vi "Display Channel Datapath.vi"(0 "llp packet":T5, 1 "reset":bool, 2 "clear processing pipeline":bool, 3 "gate display until frame complete":bool, 5 "serial channel display parameters":T9, 7 "serial channel selector":fxp<+,3,3>, 9 "input valid":bool, 11 "display channel resources":T2, 12 "enable channel":bool) -> (4 "display channel status":T1, 6 "pending display frames":i8, 14 "ready for input":bool)   [LabVIEW 2020, in "GettingStarted_Common_148X_FPGA.lvlib"]
uses:
  GettingStarted_Common_148X_FPGA.lvlib
  <instrlib>/FlexRIO/CSI-2/v2/FPGA/Types/Display Parameters.ctl
  <instrlib>/FlexRIO/CSI-2/v2/Common/Types/LLP Data Type.ctl
  <instrlib>/FlexRIO/CSI-2/v2/FPGA/Types/LLP Packet.ctl
  <instrlib>/FlexRIO/CSI-2/v2/FPGA/Types/LLP Packet Header.ctl
  <instrlib>/FlexRIO/CSI-2/v2/FPGA/Types/LLP Packet Payload.ctl
  <instrlib>/FlexRIO/CSI-2/v2/FPGA/Types/LLP Packet Footer.ctl
  Types/Display Channel Resources.ctl
  Types/Serial Channel Resources.ctl
  Types/Single Serial Channel Resources.ctl
  Types/Display Channel Status.ctl
  Types/Image Metadata.ctl
  <instrlib>/FlexRIO/CSI-2/v2/FPGA/NI CSI-2 API FPGA v2.lvlib
  <instrlib>/FlexRIO/CSI-2/v2/Common/NI CSI-2 API Common v2.lvlib
  <instrlib>/_niInstr/Basic Elements/v1/FPGA/niInstr Basic Elements v1 FPGA.lvlib
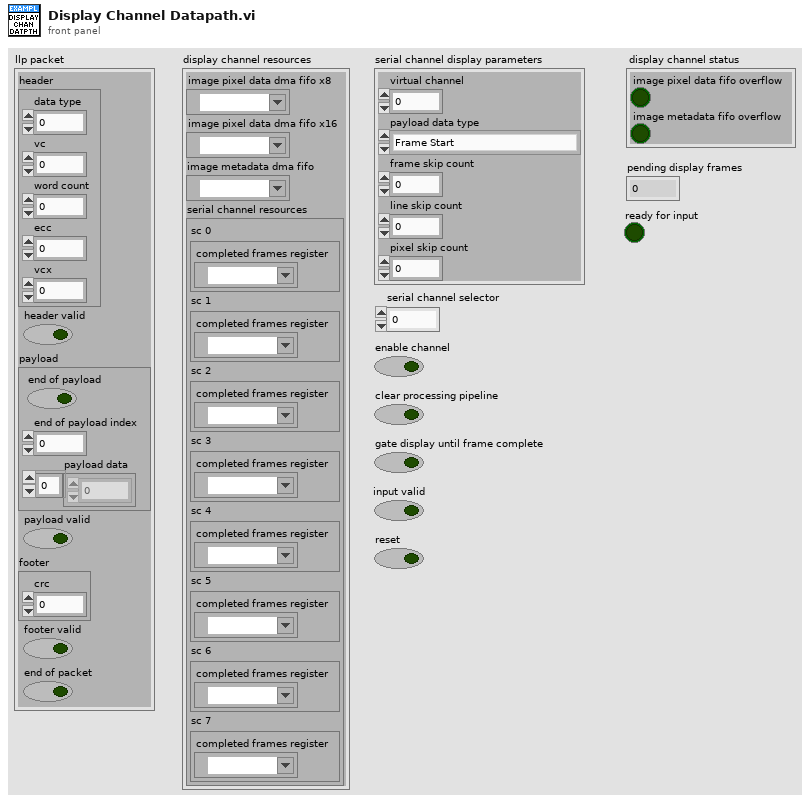
[diagram p1: front panel]
types:
  T1 = typedef "GettingStarted_Common_148X_FPGA.lvlib/Display Channel Status.ctl" = cluster{"image pixel data fifo overflow":bool, "image metadata fifo overflow":bool}
  T2 = typedef "GettingStarted_Common_148X_FPGA.lvlib/Display Channel Resources.ctl" = cluster{"image pixel data dma fifo x8":refnum<k21>, "image pixel data dma fifo x16":refnum<k21>, "image metadata dma fifo":refnum<k21>, "serial channel resources":T3}
  T3 = typedef "GettingStarted_Common_148X_FPGA.lvlib/Serial Channel Resources.ctl" = cluster{"sc 0":T4, "sc 1":T4, "sc 2":T4, "sc 3":T4, "sc 4":T4, "sc 5":T4, "sc 6":T4, "sc 7":T4}
  T4 = typedef "GettingStarted_Common_148X_FPGA.lvlib/Single Serial Channel Resources.ctl" = cluster{"completed frames register":refnum<k21>}
  T5 = typedef "NI CSI-2 API FPGA v2.lvlib/LLP Packet.ctl" = cluster{"header":T6, "header valid":bool, "payload":T7, "payload valid":bool, "footer":T8, "footer valid":bool, "end of packet":bool}
  T6 = typedef "NI CSI-2 API FPGA v2.lvlib/LLP Packet Header.ctl" = cluster{"word count":u16, "ecc":fxp<+,6,6>, "vcx":fxp<+,2,2>, "data type":fxp<+,6,6>, "vc":fxp<+,2,2>}
  T7 = typedef "NI CSI-2 API FPGA v2.lvlib/LLP Packet Payload.ctl" = cluster{"end of payload":bool, "end of payload index":fxp<+,3,3>, "payload data":u8[]}
  T8 = typedef "NI CSI-2 API FPGA v2.lvlib/LLP Packet Footer.ctl" = cluster{"crc":u16}
  T9 = typedef "NI CSI-2 API FPGA v2.lvlib/Display Parameters.ctl" = cluster{"virtual channel":fxp<+,4,4>, "payload data type":T10, "frame skip count":u16, "line skip count":u8, "pixel skip count":fxp<+,5,5>}
  T10 = typedef "NI CSI-2 API Common v2.lvlib/LLP Data Type.ctl" = enum8{"Frame Start", "Frame End", "Line Start", "Line End", "End of Transmission", "Reserved 0", "Reserved 1", "Reserved 2", "Generic Short Packet 1", "Generic Short Packet 2", "Generic Short Packet 3", "Generic Short Packet 4", "Generic Short Packet 5", "Generic Short Packet 6", "Generic Short Packet 7", "Generic Short Packet 8", "Null", "Blanking Data", "Embedded 8-bit non Image Data", "Generic Long Packet 1", "Generic Long Packet 2", "Generic Long Packet 3", "Generic Long Packet 4", "Reserved 3", "YUV420 8-bit", "YUV420 10-bit", "Legacy YUV420 8-bit", "Reserved 4", "YUV420 8-bit Chroma Shifted", "YUV420 10-bit Chroma Shifted", "YUV422 8-bit", "YUV422 10-bit", "RGB444", "RGB555", "RGB565", "RGB666", "RGB888", "Reserved 5", "Reserved 6", "RAW 24", "RAW 6", "RAW 7", "RAW 8", "RAW 10", "RAW 12", "RAW 14", "RAW 16", "RAW 20", "User Defined 8-bit Data 1", "User Defined 8-bit Data 2", "User Defined 8-bit Data 3", "User Defined 8-bit Data 4", "User Defined 8-bit Data 5", "User Defined 8-bit Data 6", "User Defined 8-bit Data 7", "User Defined 8-bit Data 8", "USL Command", "Reserved 7", "Reserved 8", "Reserved 9", "Reserved 10", "Reserved 11", "Reserved 12", "LRTE EPD Spacer"}
  T11 = typedef "GettingStarted_Common_148X_FPGA.lvlib/Image Metadata.ctl" = cluster{"serial channel":fxp<+,3,3>, "frame number":u16, "data type":T10, "width":u16, "height":u16, "image bytes":u32, "total bytes":u32, "little endian":bool}
  T12 = typedef "NI CSI-2 API FPGA v2.lvlib/Image Metadata.ctl" = cluster{"frame number":u16, "data type":T10, "width":u16, "height":u16, "image bytes":u32, "total bytes":u32, "valid":bool}
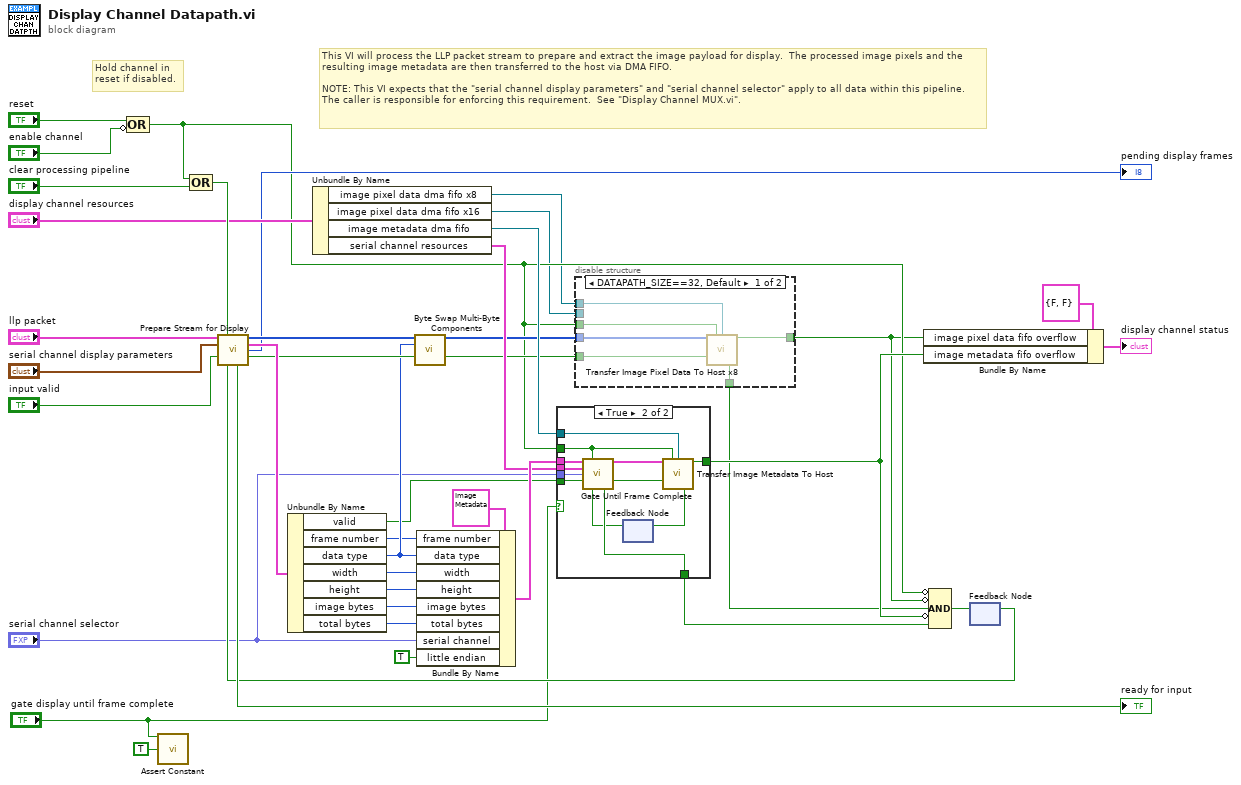
[diagram p0: block diagram]
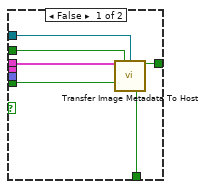
[diagram p2: hidden frame]
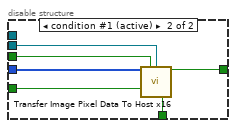
[diagram p3: hidden frame]
diagram:
  # "This VI will process the LLP packet stream to prepare and extract the image payload for display.  The processed image pixels and the resulting image metadata are then transferred to the host via DMA FIFO.\n\nNOTE: This VI expects that the \"serial channel display parameters\" and \"serial channel selector\" apply to all data within this pipeline.   The caller is responsible for enforcing this requirement.  See \"Display Channel MUX.vi\"."
  # "Hold channel in \nreset if disabled."
  n1 = Compound Arithmetic op=OR("reset", invert "enable channel") -> (w4:bool)
  n2 = call <instrlib>:"Assert Constant.vi"("constant terminal"="gate display until frame complete", "enable show error"=TRUE) -> ()  [unwired: 14 in]
  n3 = Compound Arithmetic op=OR(w4, "clear processing pipeline") -> (w18:bool)
  n4 = Unbundle By Name("display channel resources") -> ("image pixel data dma fifo x8"=w3:refnum<k21>, "image pixel data dma fifo x16"=w2:refnum<k21>, "image metadata dma fifo"=w41:refnum<k21>, "serial channel resources"=w10:T3)
  n5 = feedback #1() -> (w22:bool)  [unwired: 1 in]
  n6 = call <instrlib>:"Prepare Stream for Display.vi"("llp packet in"="llp packet", "reset"=w18, "display parameters"="serial channel display parameters", "input valid"="input valid", "ready for output"=w22) -> ("image pixel data"=w34:u8[], "image metadata"=w39:T12, "pending display frames"=→"pending display frames":i8, "image pixel data valid"=w33:bool, "ready for input"=→"ready for input":bool)  [unwired: 6 in]
  n7 = Unbundle By Name(w39) -> ("valid"=w14:bool, "frame number"=w16:u16, "data type"=w32:T10, "width"=w36:u16, "height"=w37:u16, "image bytes"=w38:u32, "total bytes"=w21:u32)
  n8 = call "Byte Swap Multi-Byte Components.vi"("image pixel data in"=w34, "data type"=w32, "input valid"=w33) -> ("image pixel data out"=w7:u8[], "output valid"=w6:bool)  [unwired: 11 in]
  n9 = Bundle By Name(cluster=T11 {"serial channel"=0.0, "frame number"=0, "data type"=enum."Frame Start", "width"=0, "height"=0, "image bytes"=0, "total bytes"=0, "little endian"=FALSE} ("image metadata"), "frame number"=w16, "data type"=w32, "width"=w36, "height"=w37, "image bytes"=w38, "total bytes"=w21, "serial channel"="serial channel selector", "little endian"=TRUE) -> (w15:T11)
  n10 = case shown="True" "gate display until frame complete" {
    tunnel: w41 -> [w47 w59]
    tunnel: [w46 w58] -> w27
    tunnel: w15 -> [w44 w57]
    tunnel: w14 -> [w43 w55]
    tunnel: w4 -> [w45 w53]
    tunnel: [w42 w52] -> w13
    tunnel: w10 -> [_ w49]
    tunnel: "serial channel selector" -> [_ w48]
    frame False {
      n11 = call "Transfer Image Metadata To Host.vi"("image metadata"=w44, "reset"=w45, "image metadata dma fifo"=w47, "input valid"=w43) -> ("overflow"=w46:bool, "ready for input"=w42:bool)  [unwired: 10 in]
    }
    frame True {
      n12 = feedback #2() -> (w50:bool)  [unwired: 1 in]
      n13 = call "Gate Until Frame Complete.vi"("image metadata in"=w57, "reset"=w53, "serial channel resources"=w49, "serial channel selector"=w48, "input valid"=w55, "ready for output"=w50) -> ("image metadata out"=w56:T11, "output valid"=w54:bool, "ready for input"=w52:bool)  [unwired: 7 in]
      n14 = call "Transfer Image Metadata To Host.vi"("image metadata"=w56, "reset"=w53, "image metadata dma fifo"=w59, "input valid"=w54) -> ("overflow"=w58:bool, "ready for input"=w51:bool)  [unwired: 10 in]
      n15 = feedback-in #2(w51) -> ()
    }
  }
  n16 = disable-structure shown="DATAPATH_SIZE==32, Default" {
    disable-tunnel: w7 -> [w65 w69]
    disable-tunnel: w6 -> [w64 w68]
    disable-tunnel: w4 -> [w63 w66]
    disable-tunnel: w3 -> [w62 _]
    disable-tunnel: [w61 w71] -> w1
    disable-tunnel: [w60 w70] -> w5
    disable-tunnel: w2 -> [_ w67]
    frame condition #0 {
      n17 = call "Transfer Image Pixel Data To Host x8.vi"("image pixel data"=w65, "reset"=w63, "image pixel data dma fifo x8"=w62, "input valid"=w64) -> ("overflow"=w61:bool, "ready for input"=w60:bool)  [unwired: 10 in]
    }
    frame condition #1 (active) {
      n18 = call "Transfer Image Pixel Data To Host x16.vi"("image pixel data"=w69, "reset"=w66, "image pixel data dma fifo x16"=w67, "input valid"=w68) -> ("overflow"=w71:bool, "ready for input"=w70:bool)  [unwired: 10 in]
    }
  }
  n19 = Bundle By Name(cluster=T1 {"image pixel data fifo overflow"=FALSE, "image metadata fifo overflow"=FALSE} ("display status"), "image pixel data fifo overflow"=w1, "image metadata fifo overflow"=w27) -> (→"display channel status":T1)
  n20 = Compound Arithmetic op=AND(invert w4, invert w1, w5, invert w27, w13) -> (w25:bool)
  n21 = feedback-in #1(w25) -> ()
